vi "Shared Options Demo.vi"() -> ()   [LabVIEW 2020]
uses:
  AutoComplete/AutoComplete/AutoComplete.lvclass/AutoComplete.ctl
  AutoComplete/Launch Autocomplete Handler.vi
  AutoComplete/AutoComplete/AutoComplete.lvclass
  AutoComplete/Shared Options/Shared Options.lvclass
panel:
  in  "B":string
  in  "A":string
  # "These inputs allow entering undefined options and start with 'degF' and 'PSI' as starting options. As new values are entered, they become suggestions in both inputs."
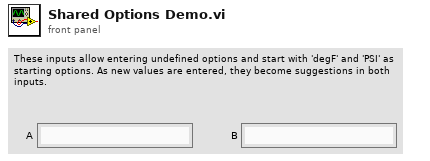
[diagram p1: front panel]
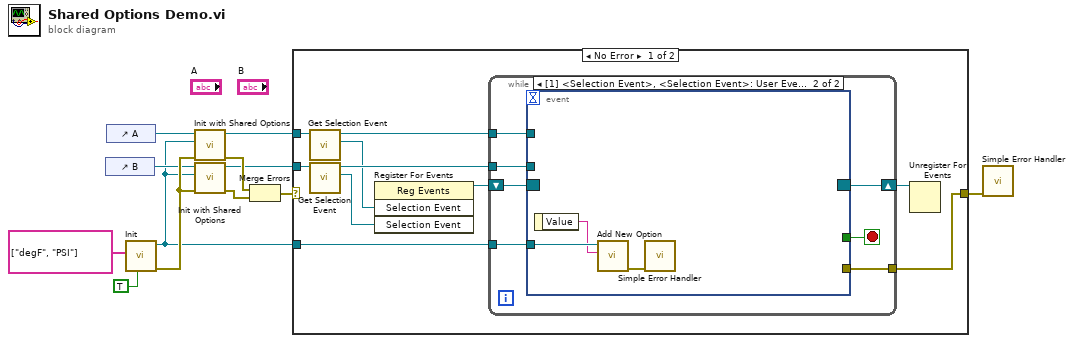
[diagram p0: block diagram]
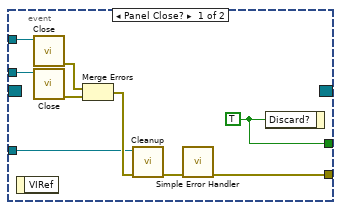
[diagram p2: hidden frame]
diagram:
  n1 = control-ref of="B"() -> (w8:refnum<vi>)
  n2 = control-ref of="A"() -> (w9:refnum<vi>)
  n3 = call "Init.vi"("Allow Undefined Values (F)"=TRUE, "Initial Options (Empty)"=string[] ["degF", "PSI"]) -> ("error out"=w11:errorcluster, "Shared Config out"=w5:refnum<class "Shared Options.lvclass">)  [unwired: 8 in]
  n4 = call "Init with Shared Options.vi"("error in (no error)"=w11, "Shared Options"=w5, "Str Refnum"=w9) -> ("error out"=w12:errorcluster, "AutoComplete out"=w7:refnum<class "AutoComplete.lvclass">)  [unwired: 7 in]
  n5 = call "Init with Shared Options.vi"("error in (no error)"=w11, "Shared Options"=w5, "Str Refnum"=w8) -> ("error out"=w4:errorcluster, "AutoComplete out"=w6:refnum<class "AutoComplete.lvclass">)  [unwired: 7 in]
  n6 = Merge Errors(w12, w4) -> (w3:errorcluster)
  n7 = case shown="No Error" w3 {
    selector: w3 -> [_ w42]
    tunnel: w7 -> [w22 _]
    tunnel: w6 -> [w21 _]
    tunnel: w5 -> [w14 _]
    tunnel: [w13 w42] -> w2
    frame No Error {
      n8 = call "Get Selection Event.vi"("AutoComplete in"=w22) -> ("Selection Event"=w18:refnum<user-event>, "AutoComplete"=w20:refnum<class "AutoComplete.lvclass">)  [unwired: 9 in]
      n9 = call "Get Selection Event.vi"("AutoComplete in"=w21) -> ("Selection Event"=w17:refnum<user-event>, "AutoComplete"=w19:refnum<class "AutoComplete.lvclass">)  [unwired: 9 in]
      n10 = register-events(w18, w17) -> (reference out=w16:refnum<event-registration>)  [unwired: 2 in, 1 out]
      n11 = while {
        tunnel: w20 -> [w24]
        tunnel: w19 -> [w25]
        shift-right: [w27] -> w15
        shift-left: w16 -> [w29]
        tunnel: w14 -> [w26]
        tunnel: [w23] -> w13
        stop <- w28 stop-if-true
        n12 = event shown="[1] <Selection Event>, <Selection Event>: User Event" {
          selector: w29 -> [_ _]
          dyn-events: [_ _] -> w27
          timeout: _ -> [_ _]
          tunnel: [w37 _] -> w28
          tunnel: w26 -> [w32 w41]
          tunnel: w25 -> [w36 _]
          tunnel: w24 -> [w35 _]
          tunnel: [w30 _] -> w23
          event Panel Close? {
            w37 = TRUE ("Discard?")
            n13 = event-data() -> ()  [unwired: 1 in, 1 out]
            n14 = call "Close.vi"("AutoComplete in"=w35) -> ("error out"=w33:errorcluster)  [unwired: 10 in]
            n15 = call "Close.vi"("AutoComplete in"=w36) -> ("error out"=w34:errorcluster)  [unwired: 10 in]
            n16 = Merge Errors(w33, w34) -> (w38:errorcluster)
            n17 = call "Cleanup.vi"("error in (no error)"=w38, "Shared Options in"=w32) -> ("error out"=w31:errorcluster)  [unwired: 9 in]
            n18 = call <vilib>:"Simple Error Handler.vi"("error in (no error)"=w31) -> ("error out"=w30:errorcluster)  [unwired: 4 in, 4 out]
            n19 = event-data("Discard?"=w37) -> ()  [unwired: 1 in, 1 out]
          }
          event User Event {
            n20 = event-data() -> ("Value"=w40:string)  [unwired: 1 in]
            n21 = call "Add New Option.vi"("New Option"=w40, "Shared Options in"=w41) -> ("error out"=w39:errorcluster)  [unwired: 8 in, 1 out]
            n22 = call <vilib>:"Simple Error Handler.vi"("error in (no error)"=w39) -> ()  [unwired: 4 in, 5 out]
          }
        }
      }
      n23 = Unregister For Events(event registration refnum=w15) -> ()  [unwired: 1 in, 1 out]
    }
    frame Error {
    }
  }
  n24 = call <vilib>:"Simple Error Handler.vi"("error in (no error)"=w2) -> ()  [unwired: 4 in, 5 out]
